vi "HEWH RLT PRAT.vi"() -> ()   [LabVIEW 2016] (continued)
            n1263 = Bundle By Name(cluster=w2990, "User Controls.Valve Ctrl.Inlet Valve B"=w2988) -> (w2989:T86)
            n1264 = call <vilib>:"Add State(s) to Queue__jki_lib_state_machine.vi"("State(s) in Front (\"\")"="Inlet Valve B" ("State(s) in Front (\"\")"), "State(s) in (\"\")"=w2992) -> ("States Out"=w2993:string)  [unwired: 13 in]
          }
          event Value Change {
            n1265 = event-data() -> ("NewVal"=w2995:T37)  [unwired: 1 in, 5 out]
            n1266 = Bundle By Name(cluster=w2997, "User Controls.Valve Ctrl.Inlet Valve C"=w2995) -> (w2996:T86)
            n1267 = call <vilib>:"Add State(s) to Queue__jki_lib_state_machine.vi"("State(s) in Front (\"\")"="Inlet Valve C" ("State(s) in Front (\"\")"), "State(s) in (\"\")"=w2999) -> ("States Out"=w3000:string)  [unwired: 13 in]
          }
          event Value Change {
            n1268 = event-data() -> ("NewVal"=w3004:T37)  [unwired: 1 in, 5 out]
            n1269 = Bundle By Name(cluster=w3003, "User Controls.Valve Ctrl.Inlet Valve D"=w3004) -> (w3002:T86)
            n1270 = call <vilib>:"Add State(s) to Queue__jki_lib_state_machine.vi"("State(s) in Front (\"\")"="Inlet Valve D" ("State(s) in Front (\"\")"), "State(s) in (\"\")"=w3006) -> ("States Out"=w3007:string)  [unwired: 13 in]
          }
          event Value Change {
            n1271 = event-data() -> ("NewVal"=w3010:T38)  [unwired: 1 in, 5 out]
            n1272 = Bundle By Name(cluster=w3011, "User Controls.Valve Ctrl.Drain Valve A"=w3010) -> (w3012:T86)
            n1273 = call <vilib>:"Add State(s) to Queue__jki_lib_state_machine.vi"("State(s) in Front (\"\")"="Drain Valve A" ("State(s) in Front (\"\")"), "State(s) in (\"\")"=w3014) -> ("States Out"=w3015:string)  [unwired: 13 in]
          }
          event Value Change {
            n1274 = event-data() -> ("NewVal"=w3017:T38)  [unwired: 1 in, 5 out]
            n1275 = Bundle By Name(cluster=w3018, "User Controls.Valve Ctrl.Drain Valve B"=w3017) -> (w3019:T86)
            n1276 = call <vilib>:"Add State(s) to Queue__jki_lib_state_machine.vi"("State(s) in Front (\"\")"="Drain Valve B" ("State(s) in Front (\"\")"), "State(s) in (\"\")"=w3021) -> ("States Out"=w3022:string)  [unwired: 13 in]
          }
          event Value Change {
            n1277 = event-data() -> ("NewVal"=w3024:T38)  [unwired: 1 in, 5 out]
            n1278 = Bundle By Name(cluster=w3025, "User Controls.Valve Ctrl.Drain Valve C"=w3024) -> (w3026:T86)
            n1279 = call <vilib>:"Add State(s) to Queue__jki_lib_state_machine.vi"("State(s) in Front (\"\")"="Drain Valve C" ("State(s) in Front (\"\")"), "State(s) in (\"\")"=w3028) -> ("States Out"=w3029:string)  [unwired: 13 in]
          }
          event Value Change {
            n1280 = event-data() -> ("NewVal"=w3031:T38)  [unwired: 1 in, 5 out]
            n1281 = Bundle By Name(cluster=w3032, "User Controls.Valve Ctrl.Drain Valve D"=w3031) -> (w3033:T86)
            n1282 = call <vilib>:"Add State(s) to Queue__jki_lib_state_machine.vi"("State(s) in Front (\"\")"="Drain Valve D" ("State(s) in Front (\"\")"), "State(s) in (\"\")"=w3035) -> ("States Out"=w3036:string)  [unwired: 13 in]
          }
          event Value Change {
            n1283 = event-data() -> ("NewVal"=w3037:T37)  [unwired: 1 in, 5 out]
            n1284 = Bundle By Name(cluster=w3039, "User Controls.Valve Ctrl.Outlet Valve A"=w3037) -> (w3038:T86)
            n1285 = call <vilib>:"Add State(s) to Queue__jki_lib_state_machine.vi"("State(s) in Front (\"\")"="Outlet Valve A" ("State(s) in Front (\"\")"), "State(s) in (\"\")"=w3041) -> ("States Out"=w3042:string)  [unwired: 13 in]
          }
          event Value Change {
            n1286 = event-data() -> ("NewVal"=w3046:T37)  [unwired: 1 in, 5 out]
            n1287 = Bundle By Name(cluster=w3045, "User Controls.Valve Ctrl.Outlet Valve B"=w3046) -> (w3044:T86)
            n1288 = call <vilib>:"Add State(s) to Queue__jki_lib_state_machine.vi"("State(s) in Front (\"\")"="Outlet Valve B" ("State(s) in Front (\"\")"), "State(s) in (\"\")"=w3048) -> ("States Out"=w3049:string)  [unwired: 13 in]
          }
          event Value Change {
            n1289 = event-data() -> ("NewVal"=w3053:T37)  [unwired: 1 in, 5 out]
            n1290 = Bundle By Name(cluster=w3052, "User Controls.Valve Ctrl.Outlet Valve C"=w3053) -> (w3051:T86)
            n1291 = call <vilib>:"Add State(s) to Queue__jki_lib_state_machine.vi"("State(s) in Front (\"\")"="Outlet Valve C" ("State(s) in Front (\"\")"), "State(s) in (\"\")"=w3055) -> ("States Out"=w3056:string)  [unwired: 13 in]
          }
          event Value Change {
            n1292 = event-data() -> ("NewVal"=w3060:T37)  [unwired: 1 in, 5 out]
            n1293 = Bundle By Name(cluster=w3059, "User Controls.Valve Ctrl.Outlet Valve D"=w3060) -> (w3058:T86)
            n1294 = call <vilib>:"Add State(s) to Queue__jki_lib_state_machine.vi"("State(s) in Front (\"\")"="Outlet Valve D" ("State(s) in Front (\"\")"), "State(s) in (\"\")"=w3062) -> ("States Out"=w3063:string)  [unwired: 13 in]
          }
          event "Clear Errors": Value Change {
            n1295 = event-data() -> ("NewVal"=w3070:bool)  [unwired: 1 in, 5 out]
            n1296 = case shown="True" w3070 {
              tunnel: ["" "Clear Errors"] -> w3068
              frame False {
              }
              frame True {
              }
            }
            n1297 = call <vilib>:"Add State(s) to Queue__jki_lib_state_machine.vi"("State(s) in Front (\"\")"=w3068, "State(s) in (\"\")"=w3067) -> ("States Out"=w3066:string)  [unwired: 13 in]
          }
          event Value Change {
            # "This is a pop-up screen to allow the\nuser to log data and save a test"
            n1298 = event-data() -> ()  [unwired: 1 in, 6 out]
            n1299 = local read "Core HEWH Data Input A"() -> (w3086:T12)
            n1300 = Unbundle By Name(w3076) -> ("Display Data (RLT).Station Label Display"=w3075:string)
            n1301 = property on="Start/Pause test" class="Bool (strict)"("DisabledEnum"=T67."Enabled" ("Disabled")) -> ()  [unwired: 2 in, 2 out]
            n1302 = local read "Station A Test Sequence"() -> (w3088:T14[])
            n1303 = Bundle By Name(cluster=T75 {"Test Fixture Hardware"={"Power "={"Yokogawa"={"WT210"={"Sample Rate (1: 0.25s)"=1, "A Range (12: 20A)"=12, "V Range (6: 600V)"=4, "Power VISA Yokogawa WT210"="WT210"}, "WT500"={"Power VISA Yokogawa WT500"="WT500", "V Range (8: 1000V)"=0, "I Range (7: 40A)"=0, "Update Rate (3: 500ms)"=2}, "WT310_2"={"Sample Rate (1: 0.25s)"=1, "A Range (12: 20A)"=11, "V Range (6: 600V)"=4, "Power VISA Yokogawa WT310_2"=""}, "WT310_3"={"Sample Rate (1: 0.25s)"=1, "A Range (12: 20A)"=11, "V Range (6: 600V)"=4, "Power VISA Yokogawa WT310_3"=""}}, "Aplus"={"Aplus IP Address"="192.168.1.101", "Remote Port"=502, "Instrument"="APLUS", "Instr Driver Revision"="1.03.0053"}, "Power Limits"={"Crest Factor"={"Upper Limit"=1.49, "Lower Limit"=1.34}, "Harmonic Content"={"Uthd"=2.0}, "Voltage"={"% Error"=2.0}, "Stability"={"<1 Watt "={"Wattage"=1.0, "Slope (mW/H)"=10.0}, ">1 Watt"={"1%Power/Hour"=1.0}}}, "Nominal Voltage"=120, "Time Limit (s)"=10800.0, "Power Variation Limit (%)"=50.0, "Power Supply"={"Chroma 61605"="CHROMA", "Use Chroma?"=FALSE}}, "Weight Scale"={"Com Options"={"IND560Scale VISA"="IND560", "IP Address"="192.168.1.50", "Remote Port"=502, "Setra Scale VISA"="COM3", "GSE 350"="GSE350"}, "Select Scale"=""}, "Flow Rates"={"Laurel Cold IP Address"="", "Laurel Hot IP Address"="34972A_2", "Hot Water Laurel VISA"="LaurelMeter_Hot", "Cold Water Laurel VISA"="LaurelMeter_Cold", "Remote Port"=0, "Laurel Communication Type"="", "Meters To Collect (Hot Cold)"="", "HOT Laurel Reference"=refnum, "COLD Laurel Reference"=refnum}, "Analog Data"={"Agilent"={"Agilent 34972_1"="34972A_1", "Agilent 34972_2"="34972A_2", "Agilent 34972_3"="34972A_3", "Agilent 34972_4"="34972A_4", "Agilent 34972_5"="34972A_5", "Agilent 34972_6"="34972A_6", "Agilent Gain"=0.0, "TC Type (K,J,T)"="", "Instrument IDN?"="", "TC Channels-List"="", "Analog Channels-List"="", "Agilent Cluster Array"=[], "TC Channels-List 2"="", "Analog Channels-List 2"=""}, "Yokogawa"={"MW100"="MW100", "Intellifaucet"=FALSE}, "Select Analog"="", "TC Coefficients"={"TC Coefficients 1"=[], "TC Coefficients 2"=[], "TC Coefficients 3"=[], "TC Coefficients 4"=[], "TC Coefficients 5"=[], "TC Coefficients 6"=[], "TC Coefficients 7"=[]}, "NI Tasks (Dryer DOE)"=["TC Temps-Module 1", "TC Temps-Module 2", "TC Temps-Module 3", "TC Temps-Module 4", "TC Temps-Module 5", "Gas and Temp-Module 6", "AC_DC Events-Module 7"], "Laurel Analog"={"Laurel IP (Water Temp)"="", "Laurel IP (Pressure)"=""}}, "ITHX-Temp Humidity"={"IP Address 1"="", "Remote Port"=0, "IP Address 2"="", "IP Address 3"=""}, "Gas Meter COM Ports"={"Gas Meter 1"="COM3", "Gas Meter 2"="COM4", "Gas Meter 3"="COM5", "Gas Meter 4"="COM6", "Gas Meter 5"="COM7", "Gas Meter 6"="COM8"}, "Barometric Pressure"={"HEISE 901A"="HEISE", "Use Barometer?"=FALSE}}, "GEA2"={"Address"=35, "Source"=228, "Viper/Hawk"=0}, "DOE Capacity Measurments"={"Weight 1"=35.0, "Model Number 1"="", "Temp 1"=0.0, "Serial Number 1"="", "Lab Number 1"="", "Lab Number 2"="", "Serial Number 2"="", "Temp 2"=0.0, "Model Number 2"="", "Weight 2"=0.0, "Lab Number 3"="", "Serial Number 3"="", "Temp 3"=0.0, "Model Number 3"="", "Weight 3"=0.0, "Lab Number 4"="", "Serial Number 4"="", "Temp 4"=0.0, "Model Number 4"="", "Weight 4"=0.0, "Capacity Measurment Output String"=[]}, "Initialize.Washer In"={"Appliance Details"={"FileVersionInfo"={"FileVersion"="", "ProductName"="", "InternalName"="", "CompanyName"="", "LegalCopyright"="", "FileDescription"=""}, "Dishwasher Info"={"Open Cup Weight (gm):"=0.0, "Auto Cup Weight (gm):"=0.0, "Detergent-Dish:"="", "Inlet Temperature-Dish:"="", "Cycle Mode-Dish:"="", "Unit Control-Dish:"="", "Manufacturer-Dish:"=""}, "Washer Info"={"Hot Water Temperature (Fahrenheit):"="", "Cold Water Temperature (Fahrenheit):"="", "Capacity (cu.ft):"=0.0, "Initial Cloth Weight:"=0.0, "Cloth Lot:"=60, "Model Family:"="", "Program Name:"="", "Cycle Selection:"="", "Wash Temperature:"="", "Rinse Temperature:"="", "Load Size:"=""}, "File Name Output Array"=[], "Calibration Output Array"=[], "Appliance Common"={"Engineer:"="", "Model Number:"="", "Serial Number:"="", "Comments:"="", "Station ID:"="", "Technician:"="", "TR Number:"="", "Lab ID:"="", "Voltage:"="", "Water Pressure (PSI):"="", "Test Date:"="", "Computer Name:"="", "IP Address:"="", "Ambient RH:"="", "Frequency:"="", "Build:"="", "Filename:"="", "Test Type:"="", "Load Run #:"=17, "Ambient Temperature (F):"="", "File Path:"=path "", "Cycles Per Year"=0}, "Water Heater"={"Heating Mode:"=""}, "Dryer"={"Heat Setting:"="", "Washer Water Temperature (60 ± 5°F):"=7, "Water Hardness (PPM):"=7, "Dryness Setting:"="", "Dryer Type:"="", "Exhaust:"="", "Drying Cycle:"="", "Load Type:"="", "Nominal Load Weight"="", "Dryer Initial IMC Data"={"Measured IMC (lbs)"=100.0, "Actual Initial RMC (%)"=7.0, "RMC (Desired %)"=5.0, "Bone Dry Wt(lbs)"=60.0, "Tolerance(%)"=0.0, "Actual Final RMC (%)"=0.0, "CEF (lbf/kWh)"=0.0, "Minimum Weight (lbf)"=0.0, "Average Weight (lbf)"=0.0, "Maximum Weight (lbf)"=0.0, "Measured IMC In Range?"=FALSE, "Moisture Reduction Factor"=55.5, "Field Use Factor"=1.04, "Empty Dryer Cold Weigth"=0.0, "Energy Standard"=enum."D2-Automatic Dryer", "Weight Cloth (lbs)"=0.0, "Relative Moisture Content (%)"=0.0, "Relative Moisture Content - Avg (%)"=0.0}}}, "Display Data (RLT)"={"Status Color"=0, "Serial Number Display"="", "Cycle Count Display"=0, "Station Label Display"="", "Current Run Start Time Display"=0.0, "Board ID Display"="", "RPM Display"=0, "Current Display"=0.0, "Current Path Display"=path "", "Saving Display"=FALSE, "Unit Type Display"=enum."", "Total Time On Display"=0.0, "UI Button"=FALSE}}} ("Washer Controls In"), "Initialize.Washer In.Display Data (RLT).Station Label Display"=w3075) -> (w3077:T75)
            n1304 = Unbundle By Name(w3086) -> ("LV Program"=w3073:T24)
            n1305 = case shown="\"HEWH\"" w3073 {
              tunnel: ["A" ("Station Input") w3102] -> w3096
              frame Default {
              }
              frame "HEWH" {
                n1306 = local read "Station"() -> (w3102:string)
              }
            }
            n1307 = local read "File Locations A"() -> (w3085:T2)
            n1308 = call "PRAT Test Setup.vi"("Station Input"=w3096, "Test Sequence Input"=w3088, "Washer Controls In"=w3077, "Filepath In"=w3085, "Error In"=w3097, "LV Program"=w3073) -> ("Cutout Delay (sec)"=w3081:dbl, "Unit Setpoint Out"=w3079:i32, "Appliance Details"=w3083:T4, "Filepath Out"=w3084:T2, "Station ID"=w3095:T25, "Log Data Output"=w3082:bool, "Final Output"=w3098:T14[], "Cancel Output"=w3091:bool, "Test Procedure"=w3074:string, "Reset Cycle Count"=w3090:bool, "New Cycle Count Out"=w3089:i32, "Error Out"=w3094:errorcluster)  [unwired: 2 in]
            n1309 = local write "Updated Cycle Count"(w3089) -> ()
            n1310 = local write "Reset Cycle Count"(w3090) -> ()
            n1311 = case shown="False" w3091 {
              tunnel: w3098 -> [w3118 _]
              tunnel: w3095 -> [w3117 _]
              tunnel: w3094 -> [w3114 w3119]
              tunnel: [w3105 w3119] -> w3093
              tunnel: w3092 -> [w3115 _]
              tunnel: w3087 -> [w3111 _]
              tunnel: w3084 -> [w3106 _]
              tunnel: w3083 -> [w3110 _]
              tunnel: w3082 -> [w3107 _]
              tunnel: w3081 -> [w3109 _]
              tunnel: w3079 -> [w3104 _]
              tunnel: w3074 -> [w3103 _]
              frame False {
                n1312 = local write "Station ID to Reset"(w3117) -> ()
                n1313 = local write "StationA Setpoint"(w3104) -> ()
                n1314 = local write "Cutout Delay A (sec)"(w3109) -> ()
                n1315 = Generate User Event(user event=w3115, event data cluster=TRUE ("event data"), error in=w3114) -> (error out=w3112:errorcluster)  [unwired: 1 in, 1 out]
                n1316 = local write "Disable Station 1"(HEWH_RLT_Station_Disable."Enable Station" ("Disable Station 1")) -> ()
                n1317 = Generate User Event(user event=w3111, event data cluster=TRUE ("event data"), error in=w3112) -> (error out=w3105:errorcluster)  [unwired: 1 in, 1 out]
                "Station A Test Sequence" <- w3118
                "Appliance Details A" <- w3110
                "Updated File Path A" <- w3106
                "Log Data Output (A)" <- w3107
                "Test Procedure" <- w3103
              }
              frame True {
              }
            }
          }
          event Value Change {
            n1318 = event-data() -> ()  [unwired: 1 in, 6 out]
            n1319 = Unbundle By Name(w3121) -> ("Display Data (RLT).Station Label Display"=w3123:string)
            n1320 = local read "Core HEWH Data Input B"() -> (w3133:T12)
            n1321 = local read "Station B Test Sequence"() -> (w3135:T14[])
            n1322 = Bundle By Name(cluster=T75 {"Test Fixture Hardware"={"Power "={"Yokogawa"={"WT210"={"Sample Rate (1: 0.25s)"=1, "A Range (12: 20A)"=12, "V Range (6: 600V)"=4, "Power VISA Yokogawa WT210"="WT210"}, "WT500"={"Power VISA Yokogawa WT500"="WT500", "V Range (8: 1000V)"=0, "I Range (7: 40A)"=0, "Update Rate (3: 500ms)"=2}, "WT310_2"={"Sample Rate (1: 0.25s)"=1, "A Range (12: 20A)"=11, "V Range (6: 600V)"=4, "Power VISA Yokogawa WT310_2"=""}, "WT310_3"={"Sample Rate (1: 0.25s)"=1, "A Range (12: 20A)"=11, "V Range (6: 600V)"=4, "Power VISA Yokogawa WT310_3"=""}}, "Aplus"={"Aplus IP Address"="192.168.1.101", "Remote Port"=502, "Instrument"="APLUS", "Instr Driver Revision"="1.03.0053"}, "Power Limits"={"Crest Factor"={"Upper Limit"=1.49, "Lower Limit"=1.34}, "Harmonic Content"={"Uthd"=2.0}, "Voltage"={"% Error"=2.0}, "Stability"={"<1 Watt "={"Wattage"=1.0, "Slope (mW/H)"=10.0}, ">1 Watt"={"1%Power/Hour"=1.0}}}, "Nominal Voltage"=120, "Time Limit (s)"=10800.0, "Power Variation Limit (%)"=50.0, "Power Supply"={"Chroma 61605"="CHROMA", "Use Chroma?"=FALSE}}, "Weight Scale"={"Com Options"={"IND560Scale VISA"="IND560", "IP Address"="192.168.1.50", "Remote Port"=502, "Setra Scale VISA"="COM3", "GSE 350"="GSE350"}, "Select Scale"=""}, "Flow Rates"={"Laurel Cold IP Address"="", "Laurel Hot IP Address"="34972A_2", "Hot Water Laurel VISA"="LaurelMeter_Hot", "Cold Water Laurel VISA"="LaurelMeter_Cold", "Remote Port"=0, "Laurel Communication Type"="", "Meters To Collect (Hot Cold)"="", "HOT Laurel Reference"=refnum, "COLD Laurel Reference"=refnum}, "Analog Data"={"Agilent"={"Agilent 34972_1"="34972A_1", "Agilent 34972_2"="34972A_2", "Agilent 34972_3"="34972A_3", "Agilent 34972_4"="34972A_4", "Agilent 34972_5"="34972A_5", "Agilent 34972_6"="34972A_6", "Agilent Gain"=0.0, "TC Type (K,J,T)"="", "Instrument IDN?"="", "TC Channels-List"="", "Analog Channels-List"="", "Agilent Cluster Array"=[], "TC Channels-List 2"="", "Analog Channels-List 2"=""}, "Yokogawa"={"MW100"="MW100", "Intellifaucet"=FALSE}, "Select Analog"="", "TC Coefficients"={"TC Coefficients 1"=[], "TC Coefficients 2"=[], "TC Coefficients 3"=[], "TC Coefficients 4"=[], "TC Coefficients 5"=[], "TC Coefficients 6"=[], "TC Coefficients 7"=[]}, "NI Tasks (Dryer DOE)"=["TC Temps-Module 1", "TC Temps-Module 2", "TC Temps-Module 3", "TC Temps-Module 4", "TC Temps-Module 5", "Gas and Temp-Module 6", "AC_DC Events-Module 7"], "Laurel Analog"={"Laurel IP (Water Temp)"="", "Laurel IP (Pressure)"=""}}, "ITHX-Temp Humidity"={"IP Address 1"="", "Remote Port"=0, "IP Address 2"="", "IP Address 3"=""}, "Gas Meter COM Ports"={"Gas Meter 1"="COM3", "Gas Meter 2"="COM4", "Gas Meter 3"="COM5", "Gas Meter 4"="COM6", "Gas Meter 5"="COM7", "Gas Meter 6"="COM8"}, "Barometric Pressure"={"HEISE 901A"="HEISE", "Use Barometer?"=FALSE}}, "GEA2"={"Address"=35, "Source"=228, "Viper/Hawk"=0}, "DOE Capacity Measurments"={"Weight 1"=35.0, "Model Number 1"="", "Temp 1"=0.0, "Serial Number 1"="", "Lab Number 1"="", "Lab Number 2"="", "Serial Number 2"="", "Temp 2"=0.0, "Model Number 2"="", "Weight 2"=0.0, "Lab Number 3"="", "Serial Number 3"="", "Temp 3"=0.0, "Model Number 3"="", "Weight 3"=0.0, "Lab Number 4"="", "Serial Number 4"="", "Temp 4"=0.0, "Model Number 4"="", "Weight 4"=0.0, "Capacity Measurment Output String"=[]}, "Initialize.Washer In"={"Appliance Details"={"FileVersionInfo"={"FileVersion"="", "ProductName"="", "InternalName"="", "CompanyName"="", "LegalCopyright"="", "FileDescription"=""}, "Dishwasher Info"={"Open Cup Weight (gm):"=0.0, "Auto Cup Weight (gm):"=0.0, "Detergent-Dish:"="", "Inlet Temperature-Dish:"="", "Cycle Mode-Dish:"="", "Unit Control-Dish:"="", "Manufacturer-Dish:"=""}, "Washer Info"={"Hot Water Temperature (Fahrenheit):"="", "Cold Water Temperature (Fahrenheit):"="", "Capacity (cu.ft):"=0.0, "Initial Cloth Weight:"=0.0, "Cloth Lot:"=60, "Model Family:"="", "Program Name:"="", "Cycle Selection:"="", "Wash Temperature:"="", "Rinse Temperature:"="", "Load Size:"=""}, "File Name Output Array"=[], "Calibration Output Array"=[], "Appliance Common"={"Engineer:"="", "Model Number:"="", "Serial Number:"="", "Comments:"="", "Station ID:"="", "Technician:"="", "TR Number:"="", "Lab ID:"="", "Voltage:"="", "Water Pressure (PSI):"="", "Test Date:"="", "Computer Name:"="", "IP Address:"="", "Ambient RH:"="", "Frequency:"="", "Build:"="", "Filename:"="", "Test Type:"="", "Load Run #:"=17, "Ambient Temperature (F):"="", "File Path:"=path "", "Cycles Per Year"=0}, "Water Heater"={"Heating Mode:"=""}, "Dryer"={"Heat Setting:"="", "Washer Water Temperature (60 ± 5°F):"=7, "Water Hardness (PPM):"=7, "Dryness Setting:"="", "Dryer Type:"="", "Exhaust:"="", "Drying Cycle:"="", "Load Type:"="", "Nominal Load Weight"="", "Dryer Initial IMC Data"={"Measured IMC (lbs)"=100.0, "Actual Initial RMC (%)"=7.0, "RMC (Desired %)"=5.0, "Bone Dry Wt(lbs)"=60.0, "Tolerance(%)"=0.0, "Actual Final RMC (%)"=0.0, "CEF (lbf/kWh)"=0.0, "Minimum Weight (lbf)"=0.0, "Average Weight (lbf)"=0.0, "Maximum Weight (lbf)"=0.0, "Measured IMC In Range?"=FALSE, "Moisture Reduction Factor"=55.5, "Field Use Factor"=1.04, "Empty Dryer Cold Weigth"=0.0, "Energy Standard"=enum."D2-Automatic Dryer", "Weight Cloth (lbs)"=0.0, "Relative Moisture Content (%)"=0.0, "Relative Moisture Content - Avg (%)"=0.0}}}, "Display Data (RLT)"={"Status Color"=0, "Serial Number Display"="", "Cycle Count Display"=0, "Station Label Display"="", "Current Run Start Time Display"=0.0, "Board ID Display"="", "RPM Display"=0, "Current Display"=0.0, "Current Path Display"=path "", "Saving Display"=FALSE, "Unit Type Display"=enum."", "Total Time On Display"=0.0, "UI Button"=FALSE}}} ("Washer Controls In"), "Initialize.Washer In.Display Data (RLT).Station Label Display"=w3123) -> (w3122:T75)
            n1323 = local read "File Locations B"() -> (w3131:T2)
            n1324 = Unbundle By Name(w3133) -> ("LV Program"=w3132:T24)
            n1325 = call "PRAT Test Setup.vi"("Station Input"="B", "Test Sequence Input"=w3135, "Washer Controls In"=w3122, "Filepath In"=w3131, "Error In"=w3145, "LV Program"=w3132) -> ("Cutout Delay (sec)"=w3127:dbl, "Unit Setpoint Out"=w3125:i32, "Appliance Details"=w3129:T4, "Filepath Out"=w3130:T2, "Station ID"=w3141:T25, "Log Data Output"=w3128:bool, "Final Output"=w3144:T14[], "Cancel Output"=w3142:bool, "Test Procedure"=w3120:string, "Reset Cycle Count"=w3137:bool, "New Cycle Count Out"=→"Updated Cycle Count":i32, "Error Out"=w3140:errorcluster)  [unwired: 2 in]
            n1326 = local write "Reset Cycle Count"(w3137) -> ()
            n1327 = case shown="False" w3142 {
              tunnel: w3144 -> [w3163 _]
              tunnel: w3141 -> [w3162 _]
              tunnel: w3140 -> [w3159 w3164]
              tunnel: [w3156 w3164] -> w3139
              tunnel: w3138 -> [w3161 _]
              tunnel: w3134 -> [w3155 _]
              tunnel: w3130 -> [w3153 _]
              tunnel: w3129 -> [w3154 _]
              tunnel: w3128 -> [w3152 _]
              tunnel: w3127 -> [w3151 _]
              tunnel: w3125 -> [w3149 _]
              tunnel: w3120 -> [w3148 _]
              frame False {
                n1328 = local write "StationB Setpoint"(w3149) -> ()
                n1329 = local write "Station ID to Reset"(w3162) -> ()
                n1330 = Generate User Event(user event=w3161, event data cluster=TRUE ("event data"), error in=w3159) -> (error out=w3157:errorcluster)  [unwired: 1 in, 1 out]
                n1331 = local write "Cutout Delay B (sec)"(w3151) -> ()
                n1332 = local write "Disable Station 2"(HEWH_RLT_Station_Disable."Enable Station" ("Disable Station 2")) -> ()
                n1333 = Generate User Event(user event=w3155, event data cluster=TRUE ("event data"), error in=w3157) -> (error out=w3156:errorcluster)  [unwired: 1 in, 1 out]
                "Station B Test Sequence" <- w3163
                "Appliance Details B" <- w3154
                "Updated File Path B" <- w3153
                "Log Data Output (B)" <- w3152
                "Test Procedure 2" <- w3148
              }
              frame True {
              }
            }
            n1334 = property on="Start/Pause test" class="Bool (strict)"("DisabledEnum"=T67."Enabled" ("Disabled")) -> ()  [unwired: 2 in, 2 out]
          }
          event Value Change {
            n1335 = event-data() -> ()  [unwired: 1 in, 6 out]
            n1336 = Unbundle By Name(w3167) -> ("Display Data (RLT).Station Label Display"=w3168:string)
            n1337 = local read "Core HEWH Data Input C"() -> (w3178:T12)
            n1338 = local read "Station C Test Sequence"() -> (w3180:T14[])
            n1339 = property on="Start/Pause test" class="Bool (strict)"("DisabledEnum"=T67."Enabled" ("Disabled")) -> ()  [unwired: 2 in, 2 out]
            n1340 = Bundle By Name(cluster=T75 {"Test Fixture Hardware"={"Power "={"Yokogawa"={"WT210"={"Sample Rate (1: 0.25s)"=1, "A Range (12: 20A)"=12, "V Range (6: 600V)"=4, "Power VISA Yokogawa WT210"="WT210"}, "WT500"={"Power VISA Yokogawa WT500"="WT500", "V Range (8: 1000V)"=0, "I Range (7: 40A)"=0, "Update Rate (3: 500ms)"=2}, "WT310_2"={"Sample Rate (1: 0.25s)"=1, "A Range (12: 20A)"=11, "V Range (6: 600V)"=4, "Power VISA Yokogawa WT310_2"=""}, "WT310_3"={"Sample Rate (1: 0.25s)"=1, "A Range (12: 20A)"=11, "V Range (6: 600V)"=4, "Power VISA Yokogawa WT310_3"=""}}, "Aplus"={"Aplus IP Address"="192.168.1.101", "Remote Port"=502, "Instrument"="APLUS", "Instr Driver Revision"="1.03.0053"}, "Power Limits"={"Crest Factor"={"Upper Limit"=1.49, "Lower Limit"=1.34}, "Harmonic Content"={"Uthd"=2.0}, "Voltage"={"% Error"=2.0}, "Stability"={"<1 Watt "={"Wattage"=1.0, "Slope (mW/H)"=10.0}, ">1 Watt"={"1%Power/Hour"=1.0}}}, "Nominal Voltage"=120, "Time Limit (s)"=10800.0, "Power Variation Limit (%)"=50.0, "Power Supply"={"Chroma 61605"="CHROMA", "Use Chroma?"=FALSE}}, "Weight Scale"={"Com Options"={"IND560Scale VISA"="IND560", "IP Address"="192.168.1.50", "Remote Port"=502, "Setra Scale VISA"="COM3", "GSE 350"="GSE350"}, "Select Scale"=""}, "Flow Rates"={"Laurel Cold IP Address"="", "Laurel Hot IP Address"="34972A_2", "Hot Water Laurel VISA"="LaurelMeter_Hot", "Cold Water Laurel VISA"="LaurelMeter_Cold", "Remote Port"=0, "Laurel Communication Type"="", "Meters To Collect (Hot Cold)"="", "HOT Laurel Reference"=refnum, "COLD Laurel Reference"=refnum}, "Analog Data"={"Agilent"={"Agilent 34972_1"="34972A_1", "Agilent 34972_2"="34972A_2", "Agilent 34972_3"="34972A_3", "Agilent 34972_4"="34972A_4", "Agilent 34972_5"="34972A_5", "Agilent 34972_6"="34972A_6", "Agilent Gain"=0.0, "TC Type (K,J,T)"="", "Instrument IDN?"="", "TC Channels-List"="", "Analog Channels-List"="", "Agilent Cluster Array"=[], "TC Channels-List 2"="", "Analog Channels-List 2"=""}, "Yokogawa"={"MW100"="MW100", "Intellifaucet"=FALSE}, "Select Analog"="", "TC Coefficients"={"TC Coefficients 1"=[], "TC Coefficients 2"=[], "TC Coefficients 3"=[], "TC Coefficients 4"=[], "TC Coefficients 5"=[], "TC Coefficients 6"=[], "TC Coefficients 7"=[]}, "NI Tasks (Dryer DOE)"=["TC Temps-Module 1", "TC Temps-Module 2", "TC Temps-Module 3", "TC Temps-Module 4", "TC Temps-Module 5", "Gas and Temp-Module 6", "AC_DC Events-Module 7"], "Laurel Analog"={"Laurel IP (Water Temp)"="", "Laurel IP (Pressure)"=""}}, "ITHX-Temp Humidity"={"IP Address 1"="", "Remote Port"=0, "IP Address 2"="", "IP Address 3"=""}, "Gas Meter COM Ports"={"Gas Meter 1"="COM3", "Gas Meter 2"="COM4", "Gas Meter 3"="COM5", "Gas Meter 4"="COM6", "Gas Meter 5"="COM7", "Gas Meter 6"="COM8"}, "Barometric Pressure"={"HEISE 901A"="HEISE", "Use Barometer?"=FALSE}}, "GEA2"={"Address"=35, "Source"=228, "Viper/Hawk"=0}, "DOE Capacity Measurments"={"Weight 1"=35.0, "Model Number 1"="", "Temp 1"=0.0, "Serial Number 1"="", "Lab Number 1"="", "Lab Number 2"="", "Serial Number 2"="", "Temp 2"=0.0, "Model Number 2"="", "Weight 2"=0.0, "Lab Number 3"="", "Serial Number 3"="", "Temp 3"=0.0, "Model Number 3"="", "Weight 3"=0.0, "Lab Number 4"="", "Serial Number 4"="", "Temp 4"=0.0, "Model Number 4"="", "Weight 4"=0.0, "Capacity Measurment Output String"=[]}, "Initialize.Washer In"={"Appliance Details"={"FileVersionInfo"={"FileVersion"="", "ProductName"="", "InternalName"="", "CompanyName"="", "LegalCopyright"="", "FileDescription"=""}, "Dishwasher Info"={"Open Cup Weight (gm):"=0.0, "Auto Cup Weight (gm):"=0.0, "Detergent-Dish:"="", "Inlet Temperature-Dish:"="", "Cycle Mode-Dish:"="", "Unit Control-Dish:"="", "Manufacturer-Dish:"=""}, "Washer Info"={"Hot Water Temperature (Fahrenheit):"="", "Cold Water Temperature (Fahrenheit):"="", "Capacity (cu.ft):"=0.0, "Initial Cloth Weight:"=0.0, "Cloth Lot:"=60, "Model Family:"="", "Program Name:"="", "Cycle Selection:"="", "Wash Temperature:"="", "Rinse Temperature:"="", "Load Size:"=""}, "File Name Output Array"=[], "Calibration Output Array"=[], "Appliance Common"={"Engineer:"="", "Model Number:"="", "Serial Number:"="", "Comments:"="", "Station ID:"="", "Technician:"="", "TR Number:"="", "Lab ID:"="", "Voltage:"="", "Water Pressure (PSI):"="", "Test Date:"="", "Computer Name:"="", "IP Address:"="", "Ambient RH:"="", "Frequency:"="", "Build:"="", "Filename:"="", "Test Type:"="", "Load Run #:"=17, "Ambient Temperature (F):"="", "File Path:"=path "", "Cycles Per Year"=0}, "Water Heater"={"Heating Mode:"=""}, "Dryer"={"Heat Setting:"="", "Washer Water Temperature (60 ± 5°F):"=7, "Water Hardness (PPM):"=7, "Dryness Setting:"="", "Dryer Type:"="", "Exhaust:"="", "Drying Cycle:"="", "Load Type:"="", "Nominal Load Weight"="", "Dryer Initial IMC Data"={"Measured IMC (lbs)"=100.0, "Actual Initial RMC (%)"=7.0, "RMC (Desired %)"=5.0, "Bone Dry Wt(lbs)"=60.0, "Tolerance(%)"=0.0, "Actual Final RMC (%)"=0.0, "CEF (lbf/kWh)"=0.0, "Minimum Weight (lbf)"=0.0, "Average Weight (lbf)"=0.0, "Maximum Weight (lbf)"=0.0, "Measured IMC In Range?"=FALSE, "Moisture Reduction Factor"=55.5, "Field Use Factor"=1.04, "Empty Dryer Cold Weigth"=0.0, "Energy Standard"=enum."D2-Automatic Dryer", "Weight Cloth (lbs)"=0.0, "Relative Moisture Content (%)"=0.0, "Relative Moisture Content - Avg (%)"=0.0}}}, "Display Data (RLT)"={"Status Color"=0, "Serial Number Display"="", "Cycle Count Display"=0, "Station Label Display"="", "Current Run Start Time Display"=0.0, "Board ID Display"="", "RPM Display"=0, "Current Display"=0.0, "Current Path Display"=path "", "Saving Display"=FALSE, "Unit Type Display"=enum."", "Total Time On Display"=0.0, "UI Button"=FALSE}}} ("Washer Controls In"), "Initialize.Washer In.Display Data (RLT).Station Label Display"=w3168) -> (w3166:T75)
            n1341 = local read "File Locations C"() -> (w3176:T2)
            n1342 = Unbundle By Name(w3178) -> ("LV Program"=w3177:T24)
            n1343 = call "PRAT Test Setup.vi"("Station Input"="C", "Test Sequence Input"=w3180, "Washer Controls In"=w3166, "Filepath In"=w3176, "Error In"=w3190, "LV Program"=w3177) -> ("Cutout Delay (sec)"=w3172:dbl, "Unit Setpoint Out"=w3170:i32, "Appliance Details"=w3174:T4, "Filepath Out"=w3175:T2, "Station ID"=w3187:T25, "Log Data Output"=w3173:bool, "Final Output"=w3189:T14[], "Cancel Output"=w3183:bool, "Test Procedure"=w3165:string, "Reset Cycle Count"=→"Reset Cycle Count":bool, "New Cycle Count Out"=w3181:i32, "Error Out"=w3186:errorcluster)  [unwired: 2 in]
            n1344 = local write "Updated Cycle Count"(w3181) -> ()
            n1345 = case shown="False" w3183 {
              tunnel: w3189 -> [w3208 _]
              tunnel: w3187 -> [w3207 _]
              tunnel: w3186 -> [w3204 w3209]
              tunnel: [w3201 w3209] -> w3185
              tunnel: w3184 -> [w3205 _]
              tunnel: w3179 -> [w3200 _]
              tunnel: w3175 -> [w3198 _]
              tunnel: w3174 -> [w3199 _]
              tunnel: w3173 -> [w3197 _]
              tunnel: w3172 -> [w3196 _]
              tunnel: w3170 -> [w3194 _]
              tunnel: w3165 -> [w3193 _]
              frame False {
                n1346 = local write "StationC Setpoint"(w3194) -> ()
                n1347 = Generate User Event(user event=w3205, event data cluster=TRUE ("event data"), error in=w3204) -> (error out=w3202:errorcluster)  [unwired: 1 in, 1 out]
                n1348 = local write "Station ID to Reset"(w3207) -> ()
                n1349 = local write "Cutout Delay C (sec)"(w3196) -> ()
                n1350 = local write "Disable Station 3"(HEWH_RLT_Station_Disable."Enable Station" ("Disable Station 3")) -> ()
                n1351 = Generate User Event(user event=w3200, event data cluster=TRUE ("event data"), error in=w3202) -> (error out=w3201:errorcluster)  [unwired: 1 in, 1 out]
                "Station C Test Sequence" <- w3208
                "Appliance Details C" <- w3199
                "Updated File Path C" <- w3198
                "Log Data Output (C)" <- w3197
                "Test Procedure 3" <- w3193
              }
              frame True {
              }
            }
          }
          event Value Change {
            n1352 = event-data() -> ()  [unwired: 1 in, 6 out]
            n1353 = Unbundle By Name(w3212) -> ("Display Data (RLT).Station Label Display"=w3213:string)
            n1354 = property on="Start/Pause test" class="Bool (strict)"("DisabledEnum"=T67."Enabled" ("Disabled")) -> ()  [unwired: 2 in, 2 out]
            n1355 = local read "Core HEWH Data Input D"() -> (w3223:T12)
            n1356 = local read "Station D Test Sequence"() -> (w3225:T14[])
            n1357 = Bundle By Name(cluster=T75 {"Test Fixture Hardware"={"Power "={"Yokogawa"={"WT210"={"Sample Rate (1: 0.25s)"=1, "A Range (12: 20A)"=12, "V Range (6: 600V)"=4, "Power VISA Yokogawa WT210"="WT210"}, "WT500"={"Power VISA Yokogawa WT500"="WT500", "V Range (8: 1000V)"=0, "I Range (7: 40A)"=0, "Update Rate (3: 500ms)"=2}, "WT310_2"={"Sample Rate (1: 0.25s)"=1, "A Range (12: 20A)"=11, "V Range (6: 600V)"=4, "Power VISA Yokogawa WT310_2"=""}, "WT310_3"={"Sample Rate (1: 0.25s)"=1, "A Range (12: 20A)"=11, "V Range (6: 600V)"=4, "Power VISA Yokogawa WT310_3"=""}}, "Aplus"={"Aplus IP Address"="192.168.1.101", "Remote Port"=502, "Instrument"="APLUS", "Instr Driver Revision"="1.03.0053"}, "Power Limits"={"Crest Factor"={"Upper Limit"=1.49, "Lower Limit"=1.34}, "Harmonic Content"={"Uthd"=2.0}, "Voltage"={"% Error"=2.0}, "Stability"={"<1 Watt "={"Wattage"=1.0, "Slope (mW/H)"=10.0}, ">1 Watt"={"1%Power/Hour"=1.0}}}, "Nominal Voltage"=120, "Time Limit (s)"=10800.0, "Power Variation Limit (%)"=50.0, "Power Supply"={"Chroma 61605"="CHROMA", "Use Chroma?"=FALSE}}, "Weight Scale"={"Com Options"={"IND560Scale VISA"="IND560", "IP Address"="192.168.1.50", "Remote Port"=502, "Setra Scale VISA"="COM3", "GSE 350"="GSE350"}, "Select Scale"=""}, "Flow Rates"={"Laurel Cold IP Address"="", "Laurel Hot IP Address"="34972A_2", "Hot Water Laurel VISA"="LaurelMeter_Hot", "Cold Water Laurel VISA"="LaurelMeter_Cold", "Remote Port"=0, "Laurel Communication Type"="", "Meters To Collect (Hot Cold)"="", "HOT Laurel Reference"=refnum, "COLD Laurel Reference"=refnum}, "Analog Data"={"Agilent"={"Agilent 34972_1"="34972A_1", "Agilent 34972_2"="34972A_2", "Agilent 34972_3"="34972A_3", "Agilent 34972_4"="34972A_4", "Agilent 34972_5"="34972A_5", "Agilent 34972_6"="34972A_6", "Agilent Gain"=0.0, "TC Type (K,J,T)"="", "Instrument IDN?"="", "TC Channels-List"="", "Analog Channels-List"="", "Agilent Cluster Array"=[], "TC Channels-List 2"="", "Analog Channels-List 2"=""}, "Yokogawa"={"MW100"="MW100", "Intellifaucet"=FALSE}, "Select Analog"="", "TC Coefficients"={"TC Coefficients 1"=[], "TC Coefficients 2"=[], "TC Coefficients 3"=[], "TC Coefficients 4"=[], "TC Coefficients 5"=[], "TC Coefficients 6"=[], "TC Coefficients 7"=[]}, "NI Tasks (Dryer DOE)"=["TC Temps-Module 1", "TC Temps-Module 2", "TC Temps-Module 3", "TC Temps-Module 4", "TC Temps-Module 5", "Gas and Temp-Module 6", "AC_DC Events-Module 7"], "Laurel Analog"={"Laurel IP (Water Temp)"="", "Laurel IP (Pressure)"=""}}, "ITHX-Temp Humidity"={"IP Address 1"="", "Remote Port"=0, "IP Address 2"="", "IP Address 3"=""}, "Gas Meter COM Ports"={"Gas Meter 1"="COM3", "Gas Meter 2"="COM4", "Gas Meter 3"="COM5", "Gas Meter 4"="COM6", "Gas Meter 5"="COM7", "Gas Meter 6"="COM8"}, "Barometric Pressure"={"HEISE 901A"="HEISE", "Use Barometer?"=FALSE}}, "GEA2"={"Address"=35, "Source"=228, "Viper/Hawk"=0}, "DOE Capacity Measurments"={"Weight 1"=35.0, "Model Number 1"="", "Temp 1"=0.0, "Serial Number 1"="", "Lab Number 1"="", "Lab Number 2"="", "Serial Number 2"="", "Temp 2"=0.0, "Model Number 2"="", "Weight 2"=0.0, "Lab Number 3"="", "Serial Number 3"="", "Temp 3"=0.0, "Model Number 3"="", "Weight 3"=0.0, "Lab Number 4"="", "Serial Number 4"="", "Temp 4"=0.0, "Model Number 4"="", "Weight 4"=0.0, "Capacity Measurment Output String"=[]}, "Initialize.Washer In"={"Appliance Details"={"FileVersionInfo"={"FileVersion"="", "ProductName"="", "InternalName"="", "CompanyName"="", "LegalCopyright"="", "FileDescription"=""}, "Dishwasher Info"={"Open Cup Weight (gm):"=0.0, "Auto Cup Weight (gm):"=0.0, "Detergent-Dish:"="", "Inlet Temperature-Dish:"="", "Cycle Mode-Dish:"="", "Unit Control-Dish:"="", "Manufacturer-Dish:"=""}, "Washer Info"={"Hot Water Temperature (Fahrenheit):"="", "Cold Water Temperature (Fahrenheit):"="", "Capacity (cu.ft):"=0.0, "Initial Cloth Weight:"=0.0, "Cloth Lot:"=60, "Model Family:"="", "Program Name:"="", "Cycle Selection:"="", "Wash Temperature:"="", "Rinse Temperature:"="", "Load Size:"=""}, "File Name Output Array"=[], "Calibration Output Array"=[], "Appliance Common"={"Engineer:"="", "Model Number:"="", "Serial Number:"="", "Comments:"="", "Station ID:"="", "Technician:"="", "TR Number:"="", "Lab ID:"="", "Voltage:"="", "Water Pressure (PSI):"="", "Test Date:"="", "Computer Name:"="", "IP Address:"="", "Ambient RH:"="", "Frequency:"="", "Build:"="", "Filename:"="", "Test Type:"="", "Load Run #:"=17, "Ambient Temperature (F):"="", "File Path:"=path "", "Cycles Per Year"=0}, "Water Heater"={"Heating Mode:"=""}, "Dryer"={"Heat Setting:"="", "Washer Water Temperature (60 ± 5°F):"=7, "Water Hardness (PPM):"=7, "Dryness Setting:"="", "Dryer Type:"="", "Exhaust:"="", "Drying Cycle:"="", "Load Type:"="", "Nominal Load Weight"="", "Dryer Initial IMC Data"={"Measured IMC (lbs)"=100.0, "Actual Initial RMC (%)"=7.0, "RMC (Desired %)"=5.0, "Bone Dry Wt(lbs)"=60.0, "Tolerance(%)"=0.0, "Actual Final RMC (%)"=0.0, "CEF (lbf/kWh)"=0.0, "Minimum Weight (lbf)"=0.0, "Average Weight (lbf)"=0.0, "Maximum Weight (lbf)"=0.0, "Measured IMC In Range?"=FALSE, "Moisture Reduction Factor"=55.5, "Field Use Factor"=1.04, "Empty Dryer Cold Weigth"=0.0, "Energy Standard"=enum."D2-Automatic Dryer", "Weight Cloth (lbs)"=0.0, "Relative Moisture Content (%)"=0.0, "Relative Moisture Content - Avg (%)"=0.0}}}, "Display Data (RLT)"={"Status Color"=0, "Serial Number Display"="", "Cycle Count Display"=0, "Station Label Display"="", "Current Run Start Time Display"=0.0, "Board ID Display"="", "RPM Display"=0, "Current Display"=0.0, "Current Path Display"=path "", "Saving Display"=FALSE, "Unit Type Display"=enum."", "Total Time On Display"=0.0, "UI Button"=FALSE}}} ("Washer Controls In"), "Initialize.Washer In.Display Data (RLT).Station Label Display"=w3213) -> (w3211:T75)
            n1358 = local read "File Locations D"() -> (w3219:T2)
            n1359 = Unbundle By Name(w3223) -> ("LV Program"=w3222:T24)
            n1360 = call "PRAT Test Setup.vi"("Station Input"="D", "Test Sequence Input"=w3225, "Washer Controls In"=w3211, "Filepath In"=w3219, "Error In"=w3235, "LV Program"=w3222) -> ("Cutout Delay (sec)"=w3217:dbl, "Unit Setpoint Out"=w3215:i32, "Appliance Details"=w3220:T4, "Filepath Out"=w3221:T2, "Station ID"=w3229:T25, "Log Data Output"=w3218:bool, "Final Output"=w3234:T14[], "Cancel Output"=w3232:bool, "Test Procedure"=w3210:string, "Reset Cycle Count"=w3227:bool, "New Cycle Count Out"=w3226:i32, "Error Out"=w3231:errorcluster)  [unwired: 2 in]
            n1361 = local write "Updated Cycle Count"(w3226) -> ()
            n1362 = local write "Reset Cycle Count"(w3227) -> ()
            n1363 = case shown="False" w3232 {
              tunnel: w3234 -> [w3253 _]
              tunnel: w3231 -> [w3249 w3254]
              tunnel: [w3246 w3254] -> w3230
              tunnel: w3229 -> [w3252 _]
              tunnel: w3228 -> [w3250 _]
              tunnel: w3224 -> [w3245 _]
